vi "led_command.vi"(0 "COMMAND":T1(ring), 1 "Channel":i32, 2 "Device Handle":u32, 5 "Mode":u32, 7 "Imax":u32=950, 9 "Iset":u32, 11 "Repeats":u32=9999, 12 "Strobe Profile":i32[][](array[numeric]), 13 "ERROR":errorcluster) -> (4 "Device Handle Out":u32, 6 "Channel Out":i32, 10 "LAST COMMAND":string, 15 "ERROR OUT":errorcluster)   [LabVIEW 2013]
uses:
  drivers/lib/Mightex_LEDDriver_SDK.dll
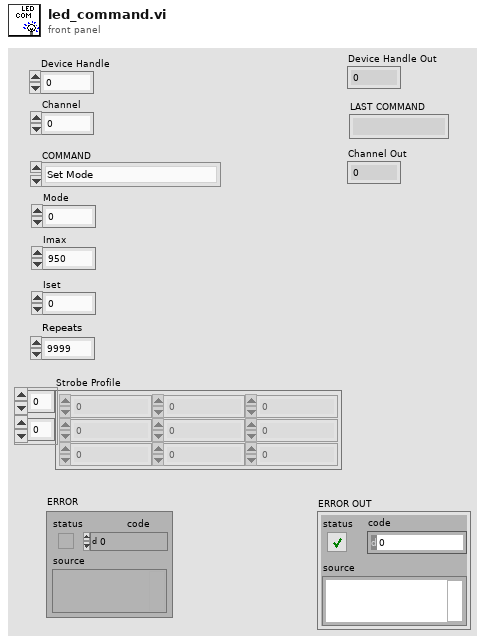
[diagram p1: front panel]
types:
  T1 = enum16{"Set Mode", "Set Normal Current ", "Set Strobe Parameters", "Set Normal Parameters", "Set Strobe Profile "}
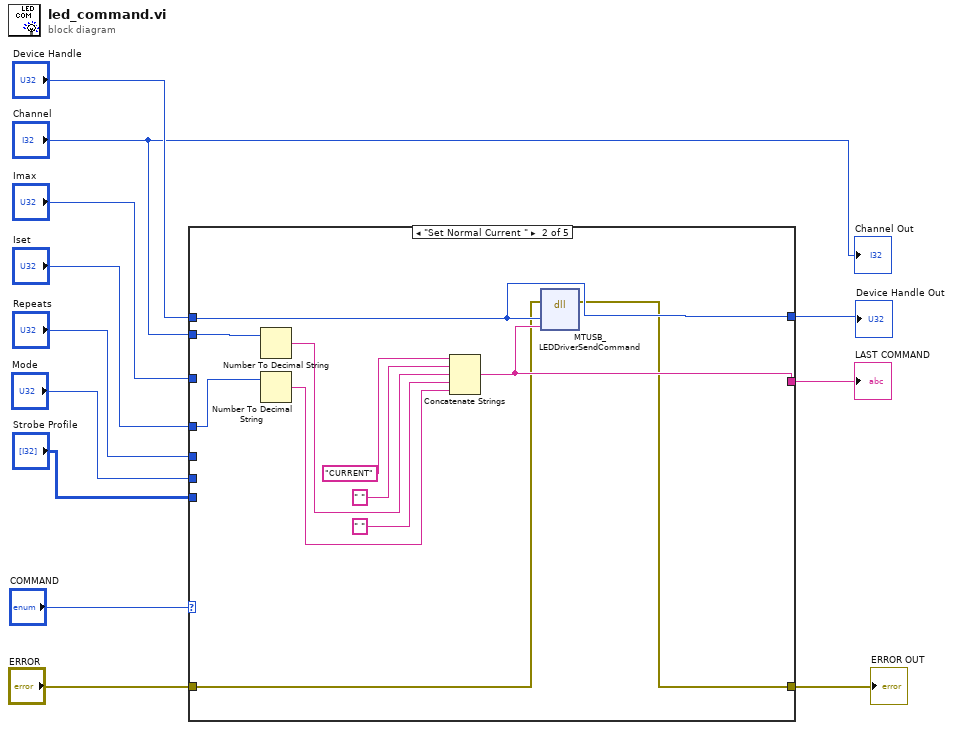
[diagram p0: block diagram]
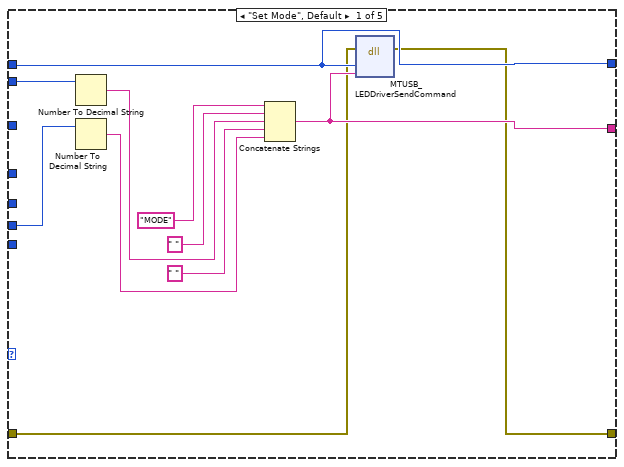
[diagram p2: hidden frame]
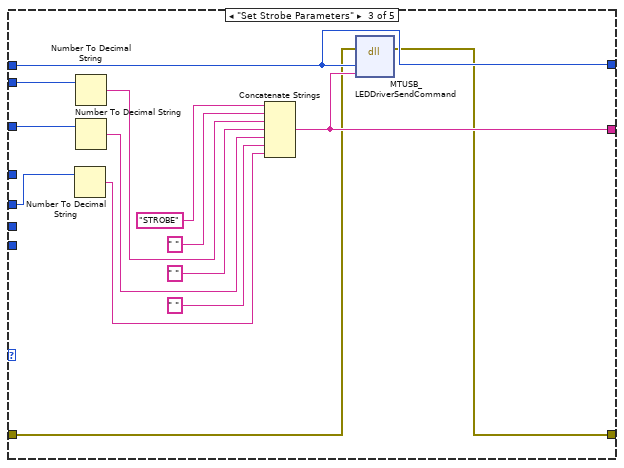
[diagram p3: hidden frame]
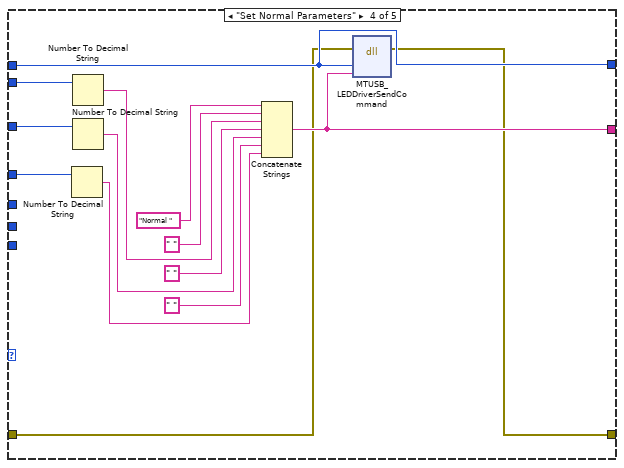
[diagram p4: hidden frame]
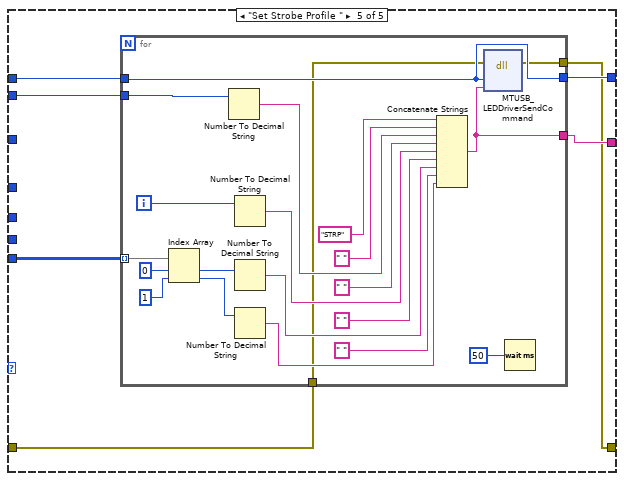
[diagram p5: hidden frame]
diagram:
  n1 = case shown="\"Set Normal Current \"" "COMMAND" {
    tunnel: "Device Handle" -> [w18 w29 w40 w53 w65]
    tunnel: "Channel" -> [w13 w25 w35 w49 w66]
    tunnel: "Imax" -> [_ _ w41 w61 _]
    tunnel: [w18 w29 w40 w53 w68] -> w10
    tunnel: [w17 w28 w39 w54 w67] -> w9
    tunnel: "Iset" -> [_ w24 _ w52 _]
    tunnel: "Repeats" -> [_ _ w38 _ _]
    tunnel: "Mode" -> [w16 _ _ _ _]
    tunnel: "Strobe Profile" -> [_ _ _ _ w69]
    tunnel: "ERROR" -> [w15 w27 w37 w51 w64]
    tunnel: [w14 w26 w36 w50 w63] -> w3
    frame "Set Mode", Default {
      n2 = Number To Decimal String(number=w13) -> (decimal integer string=w21:string)  [unwired: 1 in]
      n3 = Number To Decimal String(number=w16) -> (decimal integer string=w19:string)  [unwired: 1 in]
      n4 = Concatenate Strings("MODE", " " ("string"), w21, " " ("string"), w19) -> (w17:string)
      n5 = dll-call lib="C:/Documents and Settings/HES/Desktop/bioreactor_v2_20180123/led_control/drivers/lib/Mightex_LEDDriver_SDK.dll" fn="MTUSB_LEDDriverSendCommand"(error in=w15, "arg1"=w18, "arg2"=w17) -> (error out=w14:errorcluster)  [unwired: 5 in, 1 out]
    }
    frame "Set Normal Current " {
      n6 = Number To Decimal String(number=w25) -> (decimal integer string=w32:string)  [unwired: 1 in]
      n7 = Number To Decimal String(number=w24) -> (decimal integer string=w30:string)  [unwired: 1 in]
      n8 = Concatenate Strings("CURRENT", " " ("string"), w32, " " ("string"), w30) -> (w28:string)
      n9 = dll-call lib="C:/Documents and Settings/HES/Desktop/bioreactor_v2_20180123/led_control/drivers/lib/Mightex_LEDDriver_SDK.dll" fn="MTUSB_LEDDriverSendCommand"(error in=w27, "arg1"=w29, "arg2"=w28) -> (error out=w26:errorcluster)  [unwired: 5 in, 1 out]
    }
    frame "Set Strobe Parameters" {
      n10 = Number To Decimal String(number=w38) -> (decimal integer string=w43:string)  [unwired: 1 in]
      n11 = Number To Decimal String(number=w35) -> (decimal integer string=w46:string)  [unwired: 1 in]
      n12 = Number To Decimal String(number=w41) -> (decimal integer string=w44:string)  [unwired: 1 in]
      n13 = Concatenate Strings("STROBE", " " ("string"), w46, " " ("string"), w44, " " ("string"), w43) -> (w39:string)
      n14 = dll-call lib="C:/Documents and Settings/HES/Desktop/bioreactor_v2_20180123/led_control/drivers/lib/Mightex_LEDDriver_SDK.dll" fn="MTUSB_LEDDriverSendCommand"(error in=w37, "arg1"=w40, "arg2"=w39) -> (error out=w36:errorcluster)  [unwired: 5 in, 1 out]
    }
    frame "Set Normal Parameters" {
      n15 = Number To Decimal String(number=w52) -> (decimal integer string=w56:string)  [unwired: 1 in]
      n16 = Number To Decimal String(number=w49) -> (decimal integer string=w59:string)  [unwired: 1 in]
      n17 = Number To Decimal String(number=w61) -> (decimal integer string=w57:string)  [unwired: 1 in]
      n18 = Concatenate Strings("Normal ", " " ("string"), w59, " " ("string"), w57, " " ("string"), w56) -> (w54:string)
      n19 = dll-call lib="C:/Documents and Settings/HES/Desktop/bioreactor_v2_20180123/led_control/drivers/lib/Mightex_LEDDriver_SDK.dll" fn="MTUSB_LEDDriverSendCommand"(error in=w51, "arg1"=w53, "arg2"=w54) -> (error out=w50:errorcluster)  [unwired: 5 in, 1 out]
    }
    frame "Set Strobe Profile " {
      n20 = for {
        tunnel: w69 -> [w84] mode=indexing
        tunnel: w65 -> [w86]
        tunnel: [w86] -> w68
        tunnel: [w85] -> w67
        tunnel: w66 -> [w70]
        tunnel: w64 -> [w72]
        tunnel: [w71] -> w63
        i -> [w78]
        n21 = Index Array(array=w84, index #1=0 ("index"), index #2=1 ("index")) -> (element #1=w81:i32, element #2=w80:i32)
        n22 = Number To Decimal String(number=w70) -> (decimal integer string=w88:string)  [unwired: 1 in]
        n23 = Number To Decimal String(number=w78) -> (decimal integer string=w77:string)  [unwired: 1 in]
        n24 = Number To Decimal String(number=w81) -> (decimal integer string=w76:string)  [unwired: 1 in]
        n25 = Number To Decimal String(number=w80) -> (decimal integer string=w74:string)  [unwired: 1 in]
        n26 = Concatenate Strings("STRP", " " ("string"), w88, " " ("string"), w77, " " ("string"), w76, " " ("string"), w74) -> (w85:string)
        n27 = dll-call lib="C:/Documents and Settings/HES/Desktop/bioreactor_v2_20180123/led_control/drivers/lib/Mightex_LEDDriver_SDK.dll" fn="MTUSB_LEDDriverSendCommand"(error in=w72, "arg1"=w86, "arg2"=w85) -> (error out=w71:errorcluster)  [unwired: 5 in, 1 out]
        n28 = Wait (ms)(milliseconds to wait=u32 50) -> ()  [unwired: 1 out]
      }
    }
  }
  "Device Handle Out" <- w10
  "LAST COMMAND" <- w9
  "ERROR OUT" <- w3
  "Channel Out" <- "Channel"
